vi "Listen.vi"(8 "error in (no error)":errorcluster, 9 "Timeout":i32, 11 "Execution Profiler In":refnum<class "Execution Profiler.lvclass">) -> (0 "error out":errorcluster, 3 "Execution Profiler Out":refnum<class "Execution Profiler.lvclass">)   [LabVIEW 2020, in "Execution Profiler.lvlib" / "Execution Profiler.lvclass"]
uses:
  Execution Profiler.lvclass
  Execution Profiler View Data.ctl
  Execution Profiler.lvclass/Execution Profiler.ctl
  Execution Profiler View.vi
  Execution Profiler Result View/Execution Profiler Result View.lvclass
panel:
  in  "Case result":bool
  in  "Suite result":bool
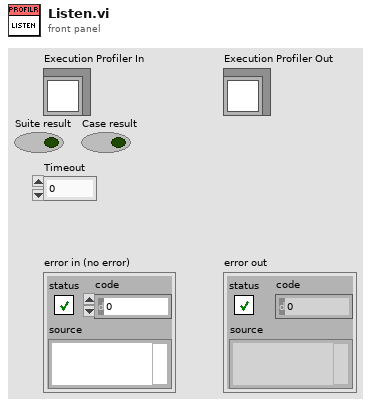
[diagram p1: front panel]
types:
  T1 = typedef "Execution Profiler.lvlib/Execution Profiler Result View.lvclass/Execution Profiler View Data.ctl" = cluster{"Timing Results":map{string, dbl}, "Tags":string[]}
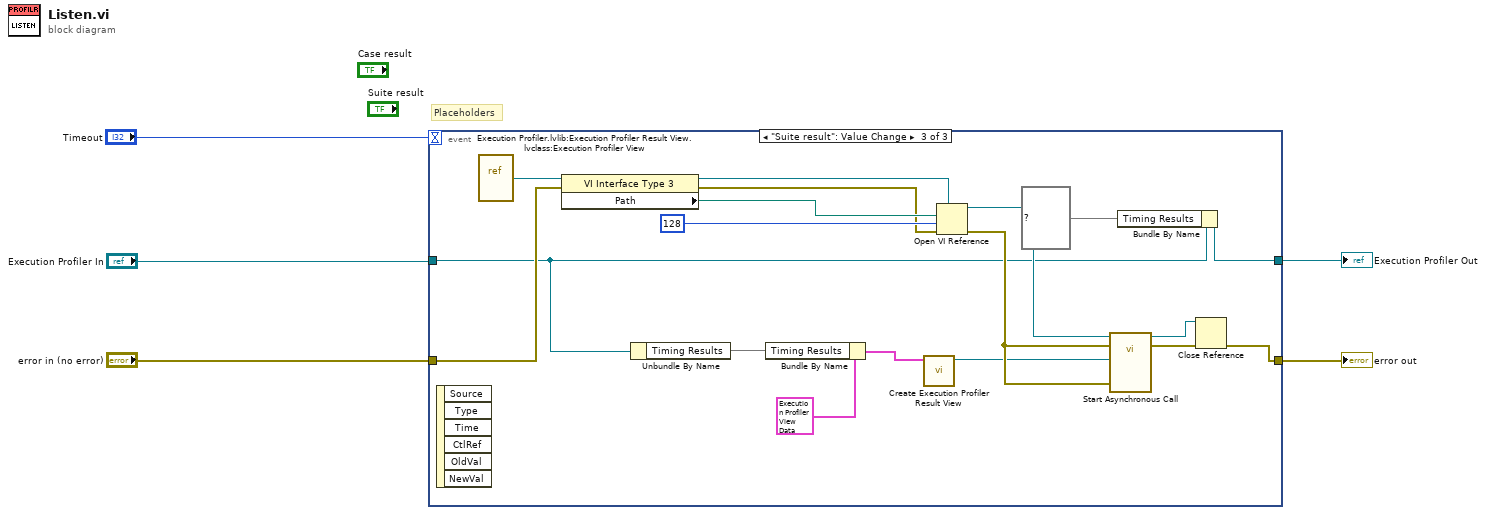
[diagram p0: block diagram]
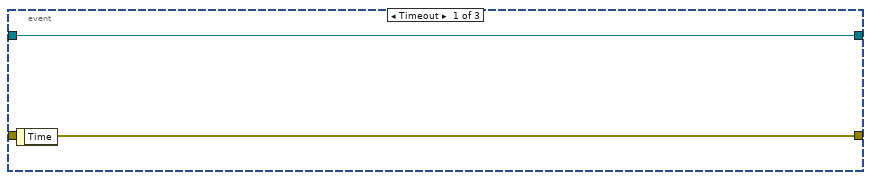
[diagram p2: hidden frame]
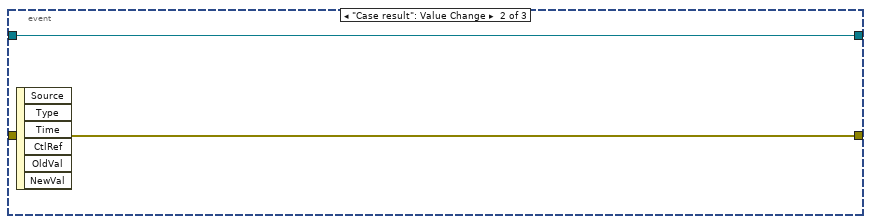
[diagram p3: hidden frame]
diagram:
  # "Placeholders"
  n1 = event shown="[2] \"Suite result\": Value Change" {
    selector: _ -> [_ _ _]
    dyn-events: _ -> [_ _ _]
    timeout: "Timeout" -> [_ _ _]
    tunnel: "error in (no error)" -> [w7 w8 w17]
    tunnel: [w7 w8 w18] -> w3
    tunnel: "Execution Profiler In" -> [w6 w9 w13]
    tunnel: [w6 w9 w16] -> w1
    event Timeout {
      n2 = event-data() -> ()  [unwired: 1 in, 1 out]
    }
    event "Case result": Value Change {
      n3 = event-data() -> ()  [unwired: 1 in, 6 out]
    }
    event "Suite result": Value Change {
      n4 = event-data() -> ()  [unwired: 1 in, 6 out]
      n5 = vi-ref "Execution Profiler.lvlib:Execution Profiler Result View.lvclass:Execution Profiler View.vi"() -> (w20:refnum<vi>)
      n6 = property class="VI Interface Type 3"(reference=w20, error in=w17) -> (reference out=w24:refnum<vi>, error out=w22:errorcluster, "Path"=w23:path)
      n7 = Unbundle By Name(w13) -> ("Timing Results"=w12:map{string, dbl})
      n8 = Bundle By Name(cluster=T1 {"Timing Results"={}, "Tags"=[]} ("Data"), "Timing Results"=w12) -> (w11:T1)
      n9 = call "Create Execution Profiler Result View.vi"("Execution Profiler Result View in"=w11) -> ("Execution Profiler Result View out"=w10:refnum<class "Execution Profiler Result View.lvclass">)  [unwired: 9 in, 1 out]
      n10 = Open VI Reference(type specifier VI Refnum (for type only)=w24, vi path=w23, options=128, error in (no error)=w22) -> (vi reference=w19:refnum<vi>, error out=w21:errorcluster)  [unwired: 2 in]
      n11 = call-by-ref "Start Asynchronous Call"(reference=w19, error in=w21, 8:"error in (no error)"=w21, "Execution Profiler Result View"=w10) -> (reference out=w27:refnum<vi>, error out=w26:errorcluster)  [unwired: 9 in, 1 out]
      n12 = Bundle By Name(cluster=w13, "Timing Results"=map{string, dbl} {}) -> (w16:refnum<class "Execution Profiler.lvclass">)
      n13 = Close Reference(reference=w27, error in (no error)=w26) -> (error out=w18:errorcluster)
    }
  }
  "error out" <- w3
  "Execution Profiler Out" <- w1
